vi "Get Unmapped Outputs.vi"(10 "module Mappings":T1, 11 "channels to module":refnum<class "TBM channel.lvclass">[](array[class])) -> (3 "unmapped outputs out":refnum<class "TBM channel.lvclass">[](array[class]))   [LabVIEW 2013, in "Engine Runtime Interface.lvclass"]
uses:
  Engine Runtime Interface.lvclass
  Engine Configuration/Module Mappings.ctl
  <vilib>/NI/Tag Bus/table/mapping specification.ctl
  <vilib>/NI/Tag Bus/tag/Data Type.ctl
  <vilib>/NI/Tag Bus/table/mapping.ctl
  <vilib>/NI/Tag Bus Module Framework/channel/TBM channel.lvclass
  <vilib>/NI/Tag Bus/tag/tag descriptor.lvclass/tag descriptor.ctl
  <vilib>/NI/Tag Bus/tag/tag descriptor.lvclass
  Engine Configuration/engine configuration.lvclass
  <vilib>/NI/Tag Bus/table/data table.lvlib
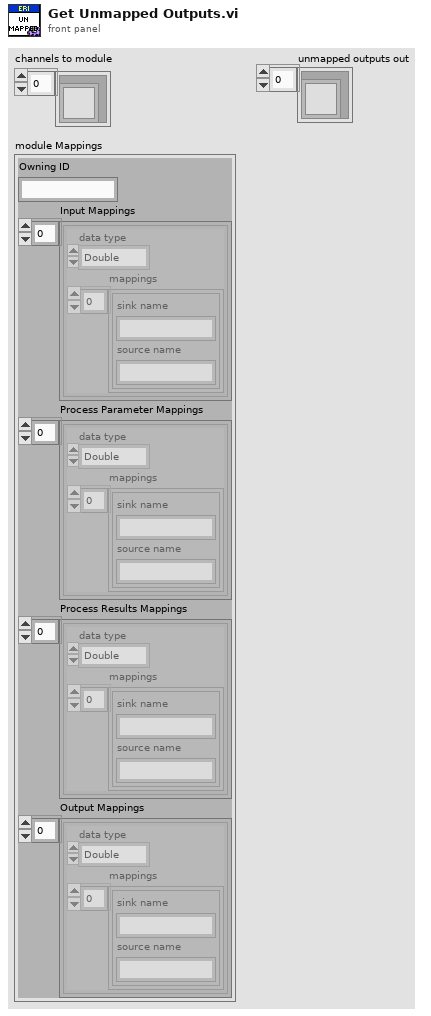
[diagram p1: front panel]
types:
  T1 = typedef "engine configuration.lvclass/Module Mappings.ctl" = cluster{"Owning ID":string, "Input Mappings":T2[], "Process Parameter Mappings":T2[], "Process Results Mappings":T2[], "Output Mappings":T2[]}
  T2 = typedef "tag bus.lvlib/data table.lvlib/mapping specification.ctl" = cluster{"data type":T3, "mappings":T4[]}
  T3 = typedef "tag bus.lvlib/tag descriptor.lvclass/Data Type.ctl" = enum16{"Double", "Single", "I64", "I32", "I16", "I8", "U64", "U32", "U16", "U8", "Boolean", "String", "Array of Double", "Array of Single", "Array of I64", "Array of I32", "Array of I16", "Array of I8", "Array of U64", "Array of U32", "Array of U16", "Array of U8", "Array of Boolean", "Array of String"}
  T4 = typedef "tag bus.lvlib/data table.lvlib/mapping.ctl" = cluster{"sink name":string, "source name":string}
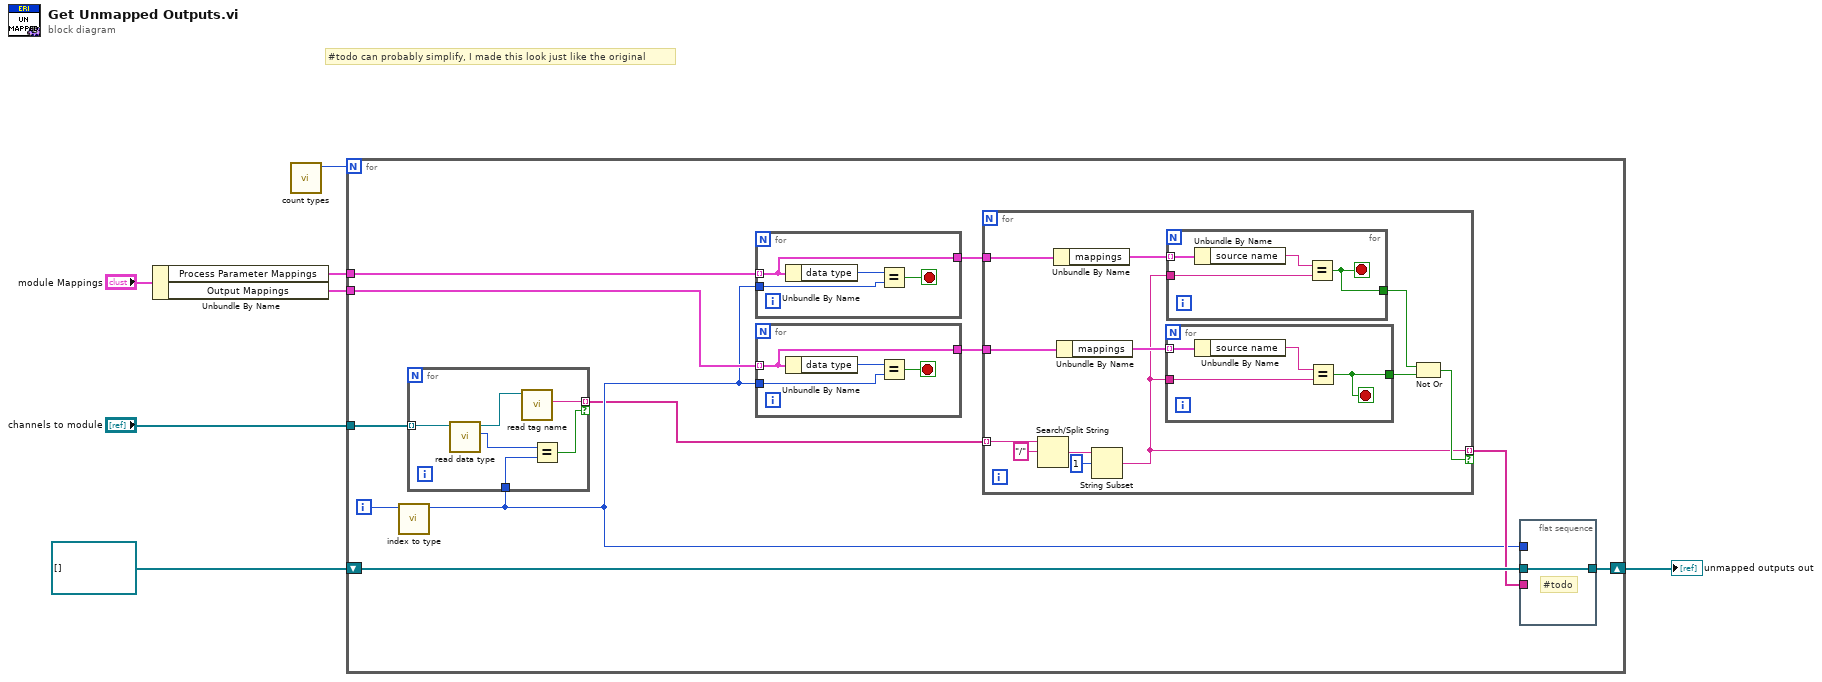
[diagram p0: block diagram]
diagram:
  # "#todo can probably simplify, I made this look just like the original"
  n1 = Unbundle By Name("module Mappings") -> ("Process Parameter Mappings"=w6:T2[], "Output Mappings"=w5:T2[])
  n2 = call <vilib>:"count types.vi"() -> ("type count"=w1:i32)  [unwired: 11 in]
  n3 = for {
    N: w1 -> [_]
    tunnel: w6 -> [w16]
    tunnel: w5 -> [w15]
    shift-right: [w12] -> w4
    shift-left: refnum<class "TBM channel.lvclass">[] [] ("channels to module") -> [w14]
    tunnel: "channels to module" -> [w11]
    i -> [w10]
    n4 = call <vilib>:"index to type.vi"("I32"=w10) -> ("type"=w9:T3)  [unwired: 10 in]
    n5 = for {
      tunnel: w11 -> [w25] mode=indexing
      tunnel: [w22] -> w8 mode=indexing if=w21
      tunnel: w9 -> [w20]
      n6 = call <vilib>:"read data type.vi"("system tag in"=w25) -> ("data type"=w23:T3, "system tag out"=w24:refnum<class "TBM channel.lvclass">)  [unwired: 8 in, 1 out]
      n7 = call <vilib>:"read tag name.vi"("system tag in"=w24) -> ("name"=w22:string)  [unwired: 8 in, 2 out]
      n8 = Equal?(x=w23, y=w20) -> (x = y?=w21:bool)
    }
    n9 = for {
      tunnel: w16 -> [w31] mode=indexing
      tunnel: [w31] -> w17
      tunnel: w9 -> [w30]
      stop <- w32 stop-if-true
      n10 = Unbundle By Name(w31) -> ("data type"=w33:T3)
      n11 = Equal?(x=w33, y=w30) -> (x = y?=w32:bool)
    }
    n12 = for {
      tunnel: w15 -> [w27] mode=indexing
      tunnel: [w27] -> w18
      tunnel: w9 -> [w26]
      stop <- w28 stop-if-true
      n13 = Unbundle By Name(w27) -> ("data type"=w29:T3)
      n14 = Equal?(x=w29, y=w26) -> (x = y?=w28:bool)
    }
    n15 = for {
      tunnel: w8 -> [w38] mode=indexing
      tunnel: w17 -> [w45]
      tunnel: w18 -> [w43]
      tunnel: [w34] -> w13 mode=indexing if=w40
      n16 = Search/Split String(string=w38, search string/char (-)="/") -> (match + rest of string=w36:string)  [unwired: 1 in, 2 out]
      n17 = Unbundle By Name(w45) -> ("mappings"=w44:T4[])
      n18 = Unbundle By Name(w43) -> ("mappings"=w42:T4[])
      n19 = String Subset(string=w36, offset (0)=1) -> (substring=w34:string)  [unwired: 1 in]
      n20 = for {
        tunnel: w42 -> [w49] mode=indexing
        tunnel: w34 -> [w47]
        tunnel: [w46] -> w41
        stop <- w46 stop-if-true
        n21 = Unbundle By Name(w49) -> ("source name"=w48:string)
        n22 = Equal?(x=w48, y=w47) -> (x = y?=w46:bool)
      }
      n23 = for {
        tunnel: w44 -> [w53] mode=indexing
        tunnel: w34 -> [w51]
        tunnel: [w50] -> w39
        stop <- w50 stop-if-true
        n24 = Unbundle By Name(w53) -> ("source name"=w52:string)
        n25 = Equal?(x=w52, y=w51) -> (x = y?=w50:bool)
      }
      n26 = Not Or(1:w41, 2:w39) -> (0:w40:bool)
    }
    n27 = flat-sequence {
      tunnel: w14 -> [w19]
      tunnel: w13 -> [_]
      tunnel: [w19] -> w12
      tunnel: w9 -> [_]
      frame #0 {
        # "#todo"
      }
    }
  }
  "unmapped outputs out" <- w4
